vi "test sv deployment.vi"() -> ()   [LabVIEW 2012]
panel:
  out "crd time":timestamp format="%<%H:%M:%S%2u>T"
  out "pas time":timestamp format="%<%H:%M:%S%2u>T"
  out "pas data":string
  out "crd data":string
  in  "stop":bool
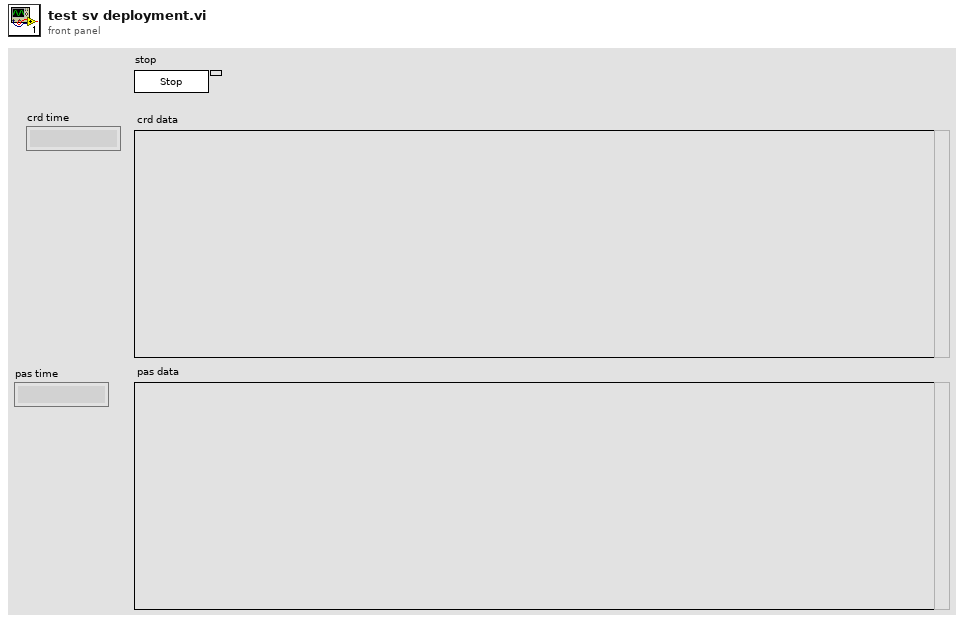
[diagram p1: front panel]
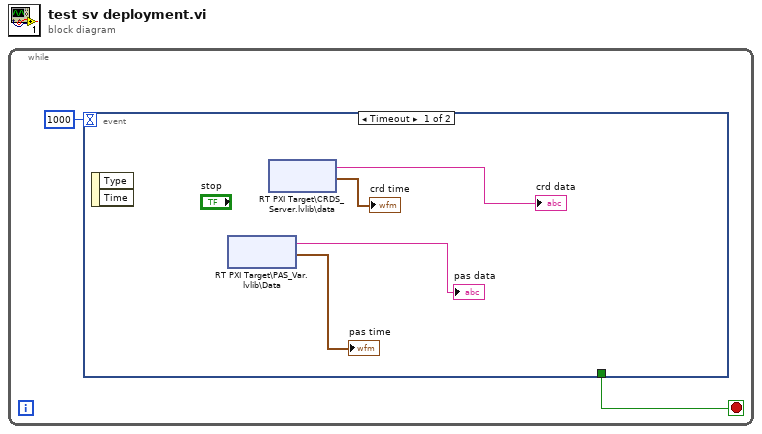
[diagram p0: block diagram]
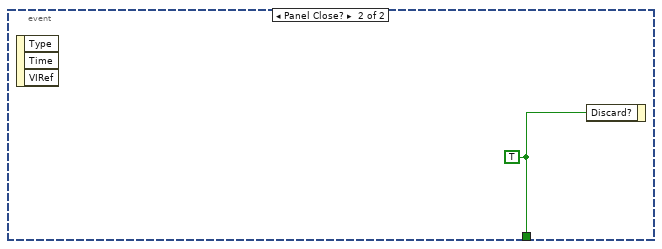
[diagram p2: hidden frame]
diagram:
  n1 = while {
    stop <- w2 stop-if-true
    n2 = event shown="[0] Timeout" {
      selector: _ -> [_ _]
      dyn-events: _ -> [_ _]
      timeout: 1000 -> [_ _]
      tunnel: [_ w7] -> w2
      event Timeout {
        n3 = event-data() -> ()  [unwired: 1 in, 2 out]
        n4 = shared-variable "RT PXI Target\\PAS_Var.lvlib\\Data"() -> (→"pas data":string, →"pas time":timestamp)  [unwired: 1 in, 1 out]
        n5 = shared-variable "RT PXI Target\\CRDS_Server.lvlib\\data"() -> (→"crd data":string, →"crd time":timestamp)  [unwired: 1 in, 1 out]
      }
      event Panel Close? {
        w7 = TRUE
        n6 = event-data() -> ()  [unwired: 1 in, 3 out]
        n7 = event-data("Discard?"=w7) -> ()  [unwired: 1 in, 1 out]
      }
    }
  }
